vi "START_STOP_2_FILE.vi"(8 "stop_y":i32, 9 "stop_x":i32, 10 "Template":path, 11 "MAP":path) -> (3 "Image":T1(plugin-control))   [LabVIEW 2015]
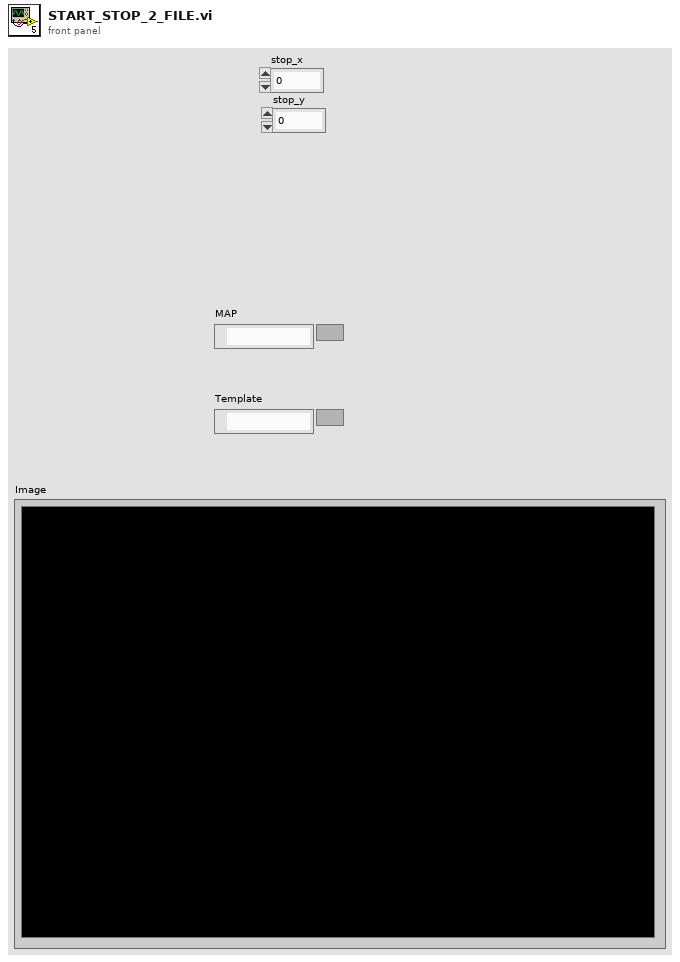
[diagram p1: front panel]
types:
  T1 = typedef "IMAQ Image.ctl" = refnum<image>
  T2 = enum16{"open", "replace", "create", "open or create", "replace or create", "replace or create with confirmation"}
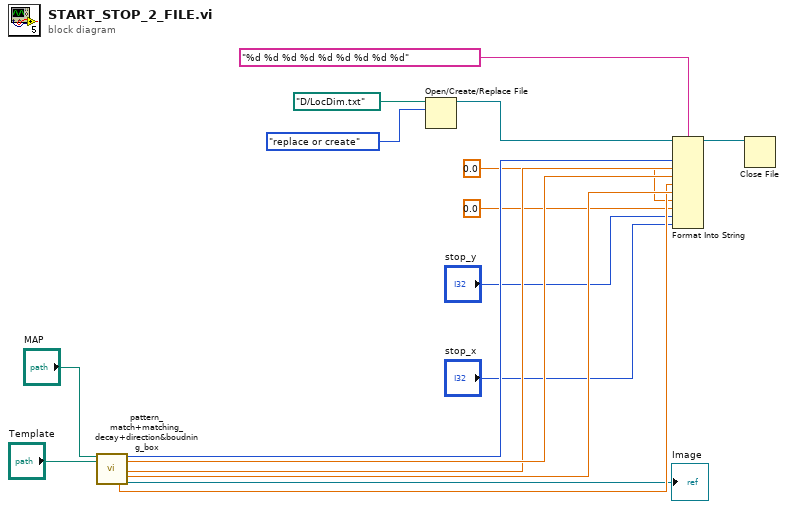
[diagram p0: block diagram]
diagram:
  n1 = call "pattern_match+matching_decay+direction&boudning_box.vi"("Imaginea"="MAP", "Template"="Template") -> ("y 2"=w9:sgl, "Directia"=w16:i32, "x"=w8:sgl, "y"=w7:sgl, "x 2"=w10:sgl, "Image"=→"Image":T1)  [unwired: 12 in]
  n2 = Open/Create/Replace File(file path (use dialog)=path "D:/LocDim.txt", operation (0:open)=T2."replace or create") -> (refnum out=w13:refnum<file>)  [unwired: 4 in, 2 out]
  n3 = Format Into String(format string="%d %d %d %d %d %d %d %d %d", initial string=w13, w16, w7, w8, w9, w10, sgl 0.0 ("input 6"), sgl 0.0 ("input 7"), "stop_y", "stop_x") -> (resulting string=w11:refnum<file>)  [unwired: 1 in, 1 out]
  n4 = Close File(refnum=w11) -> ()  [unwired: 1 in, 2 out]
